vi "MNK_Z_Bridge to PGSQL.vi"(8 "error in (no error)":errorcluster, 9 "calibration string":string, 10 "description string":string, 11 "dbl":dbl[](array[numeric])) -> (0 "error out":errorcluster)   [LabVIEW 2016]
panel:
  # "MNK Impedence Bridge to PGSQL"
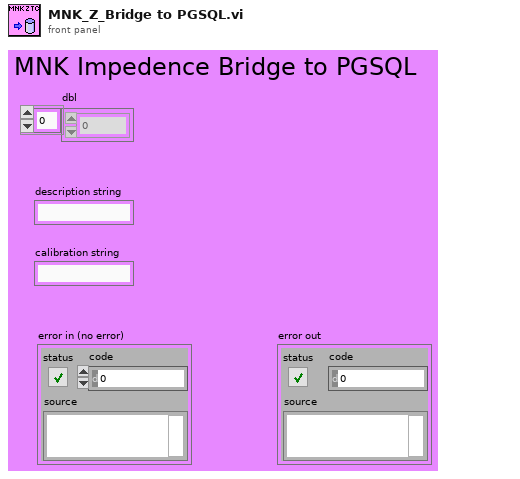
[diagram p1: front panel]
types:
  T1 = cluster{"dbl":dbl[], "description string":string, "calibration string":string}
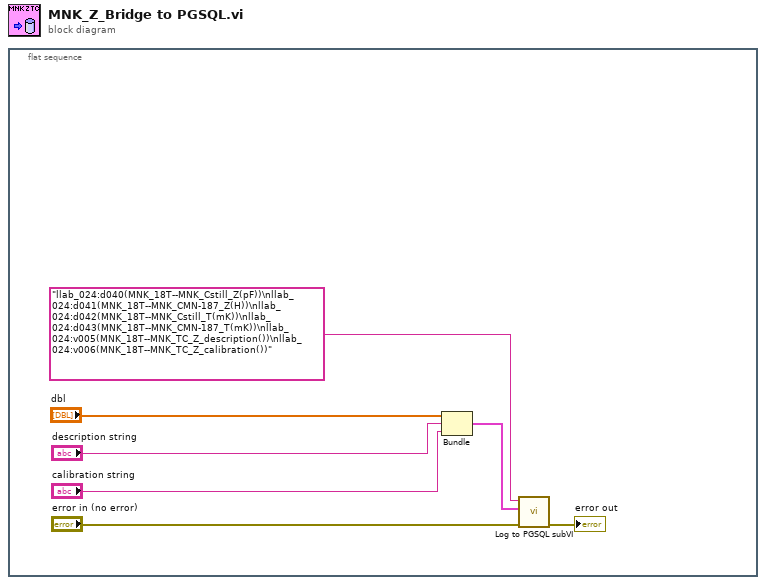
[diagram p0: block diagram]
diagram:
  n1 = flat-sequence {
    frame #0 {
      n2 = Bundle("dbl"="dbl", "description string"="description string", "calibration string"="calibration string") -> (w3:T1)  [unwired: 1 in]
      n3 = call "Log to PGSQL subVI.vi"("error in (no error)"="error in (no error)", "Data"=w3, "paths"="llab_024:d040(MNK_18T--MNK_Cstill_Z(pF))\nllab_024:d041(MNK_18T--MNK_CMN-187_Z(H))\nllab_024:d042(MNK_18T--MNK_Cstill_T(mK))\nllab_024:d043(MNK_18T--MNK_CMN-187_T(mK))\nllab_024:v005(MNK_18T--MNK_TC_Z_description())\nllab_024:v006(MNK_18T--MNK_TC_Z_calibration())") -> ("error out"=→"error out":errorcluster)  [unwired: 8 in]
    }
  }
